vi "ArmIncrementXZ.vi"(9 "AddZ":dbl, 11 "AddX":dbl) -> ()   [LabVIEW 2020]
doc: "Increment X,Y,Z values\n\nInput:\n--AddX--Double--how much to increment X\n--AddY--Double--how much to increment Y\n--AddZ--Double--how much to increment Z"
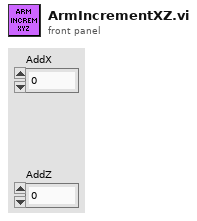
[diagram p1: front panel]
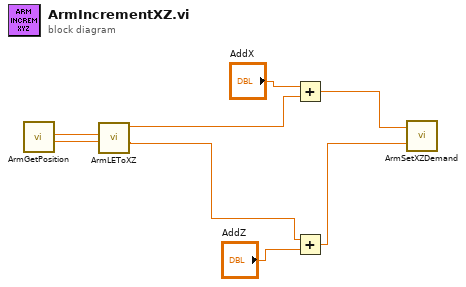
[diagram p0: block diagram]
diagram:
  n1 = call "ArmGetPosition.vi"() -> ("ExtendPostion"=w3:dbl, "LiftPostion"=w4:dbl)  [unwired: 10 in]
  n2 = call "ArmLEToXZ.vi"("Extend"=w3, "Lift"=w4) -> ("z"=w1:dbl, "x"=w2:dbl)  [unwired: 8 in]
  n3 = Add(x="AddX", y=w2) -> (x+y=w6:dbl)
  n4 = Add(x=w1, y="AddZ") -> (x+y=w5:dbl)
  n5 = call "ArmSetXZDemand.vi"("SetZ"=w5, "SetX"=w6) -> ()  [unwired: 10 in]
